vi "Exercise 3.vi"() -> ()   [LabVIEW 2017]
panel:
  out "Kelvin":dbl(slide) scale=0.0..500.0
  out "Fahrenheit":dbl(slide) scale=0.0..200.0
  in  "Celcius":dbl(slide) scale=0.0..50.0
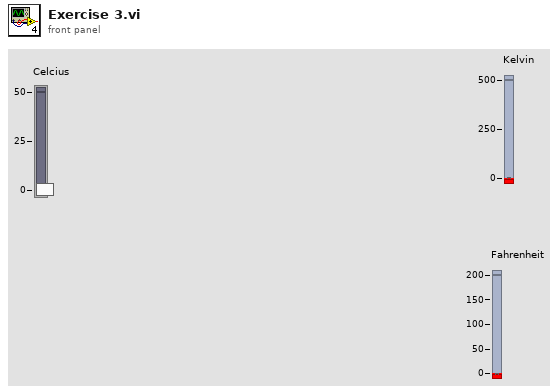
[diagram p1: front panel]
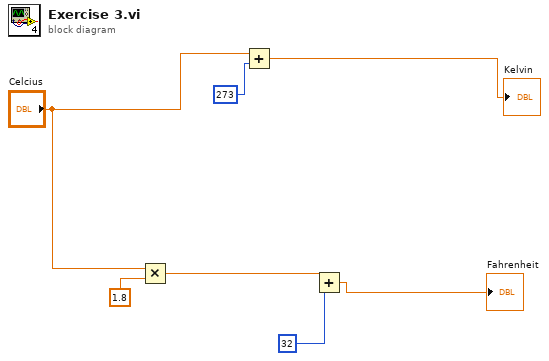
[diagram p0: block diagram]
diagram:
  n1 = Multiply(x="Celcius", y=1.8) -> (x*y=w6:dbl)
  n2 = Add(x="Celcius", y=273) -> (x+y=→"Kelvin":dbl)
  n3 = Add(x=32, y=w6) -> (x+y=→"Fahrenheit":dbl)
